vi "OP30_VERIFY_STN_12_32_25_PM.vi"() -> ()   [LabVIEW 2020]
panel:
  in  "OP30_VERIFY_STN":T1
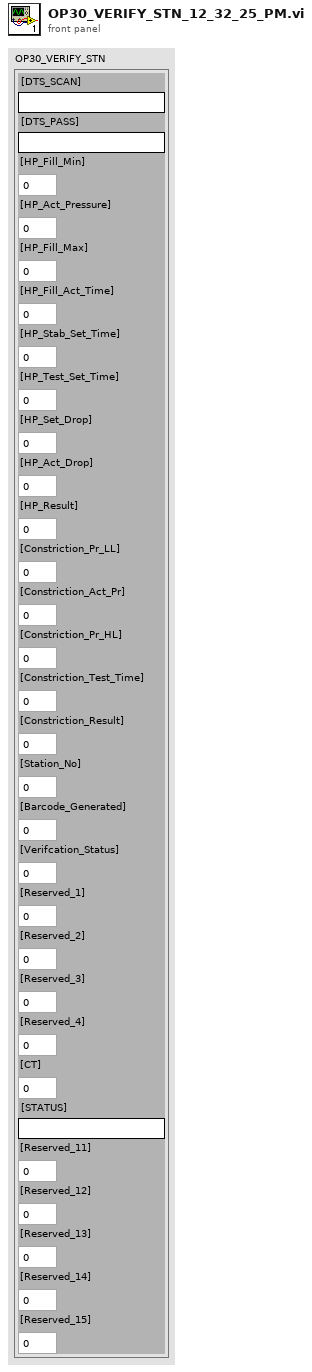
[diagram p1: front panel]
types:
  T1 = cluster{"[DTS_SCAN]":string, "[DTS_PASS]":string, "[HP_Fill_Min]":dbl, "[HP_Act_Pressure]":dbl, "[HP_Fill_Max]":dbl, "[HP_Fill_Act_Time]":dbl, "[HP_Stab_Set_Time]":dbl, "[HP_Test_Set_Time]":dbl, "[HP_Set_Drop]":dbl, "[HP_Act_Drop]":dbl, "[HP_Result]":dbl, "[Constriction_Pr_LL]":dbl, "[Constriction_Act_Pr]":dbl, "[Constriction_Pr_HL]":dbl, "[Constriction_Test_Time]":dbl, "[Constriction_Result]":dbl, "[Station_No]":dbl, "[Barcode_Generated]":dbl, "[Verifcation_Status]":dbl, "[Reserved_1]":dbl, "[Reserved_2]":dbl, "[Reserved_3]":dbl, "[Reserved_4]":dbl, "[CT]":dbl, "[STATUS]":string, "[Reserved_11]":dbl, "[Reserved_12]":dbl, "[Reserved_13]":dbl, "[Reserved_14]":dbl, "[Reserved_15]":dbl}
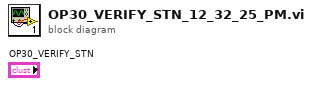
[diagram p0: block diagram]
diagram:
